vi "Write_parameter.vi"(8 "error in (no error)":errorcluster caption="entrée d'erreur (pas d'erreur)", 10 "Parameter":string, 11 "Class Instrument Firebase Altyor en entrée":refnum<class "Class Instrument Database Altyor.lvclass">) -> (0 "error out":errorcluster caption="sortie d'erreur", 3 "Class Instrument Firebase Altyor en sortie":refnum<class "Class Instrument Database Altyor.lvclass">)   [LabVIEW 2020, in "Library Instrument & Equipement.lvlib" / "Library Instruments.lvlib" / "Class Instrument Database Altyor.lvclass"]
uses:
  Class Instrument Database Altyor.lvclass
  Database/Database Altyor/Database Altyor.lvclass
  JSON API/JSON Value/Set from JSON string.vi
  Instrument (Default)/Class Instrument (Default).lvclass
  JSON API/JSON Value/JSON Value.lvclass
  JSON API/Variant JSON/Variant JSON.lvlib
  JSON API/Get Polymorphic/JSON GetSet.lvlib
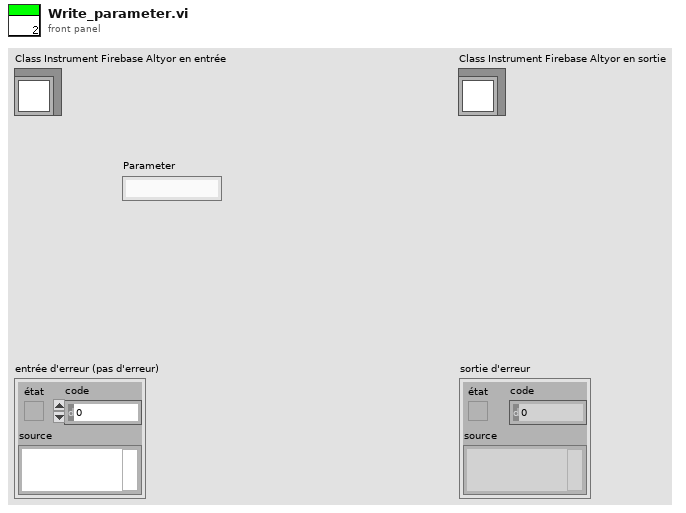
[diagram p1: front panel]
types:
  T1 = cluster{"Connection Name ODBC":string, "DatabaseName":string, "Condition":string, "Type Data ":enum16{"Data Product", "Data Test"}, "Database Altyor":refnum<class "Database Altyor.lvclass">}
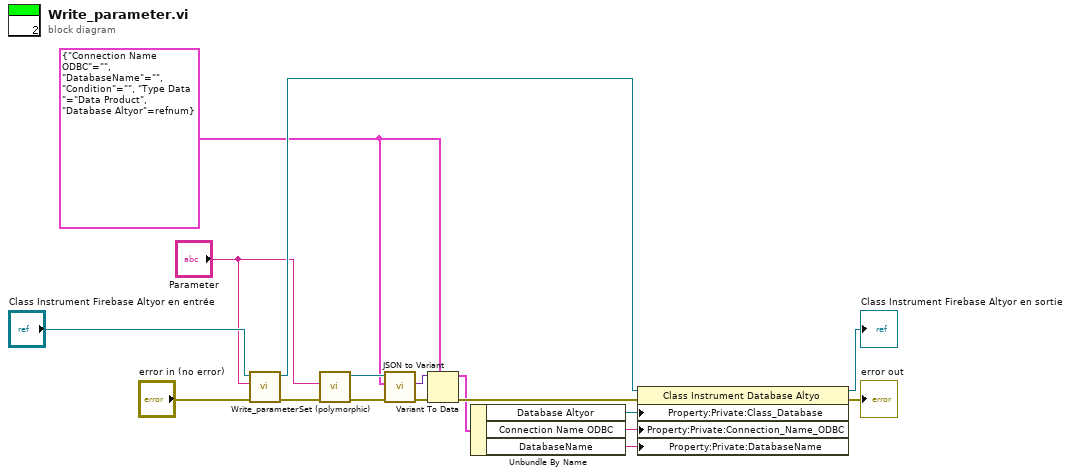
[diagram p0: block diagram]
diagram:
  w2 = T1 {"Connection Name ODBC"="", "DatabaseName"="", "Condition"="", "Type Data "=enum."Data Product", "Database Altyor"=refnum} ("Parameter")
  n1 = call-parent "Write_parameter.vi"("error in (no error)"="error in (no error)", "Parameter"="Parameter", "Class Instrument (Default) en entrée"="Class Instrument Firebase Altyor en entrée") -> ("error out"=w6:errorcluster, "Class Instrument (Default) en sortie"=w4:refnum<class "Class Instrument Database Altyor.lvclass">)  [unwired: 7 in]
  n2 = call-poly "Set (polymorphic).vi"("error in (no error)"=w6, "JSON stream"="Parameter") -> ("error out"=w15:errorcluster, "JSON Value out"=w17:refnum<class "JSON Value.lvclass">)  [unwired: 7 in, 1 out]
  n3 = call "JSON to Variant.vi"("error in (no error)"=w15, "Variant (Data Type)"=w2, "JSON Value"=w17) -> ("error out"=w16:errorcluster, "Variant out"=w14:variant)  [unwired: 7 in]
  n4 = Variant To Data(error in=w16, type=w2, Variant=w14) -> (data=w9:T1, error out=w11:errorcluster)
  n5 = Unbundle By Name(w9) -> ("Database Altyor"=w8:refnum<class "Database Altyor.lvclass">, "Connection Name ODBC"=w7:string, "DatabaseName"=w1:string)
  n6 = property class="Class Instrument Database Altyo"(reference=w4, error in=w11, "Property:Private:Class_Database"=w8, "Property:Private:Connection_Name_ODBC"=w7, "Property:Private:DatabaseName"=w1) -> (reference out=→"Class Instrument Firebase Altyor en sortie":refnum<class "Class Instrument Database Altyor.lvclass">, error out=→"error out":errorcluster)
